vi "NTV_AutoStringArray.vi"(7 "Read(f) Write(t)":bool, 11 "Array":string[](array[string])) -> (3 "Array 2":string[](array[string]))   [LabVIEW 2020]
uses:
  <vilib>/Rock Robotics/Network Tables/NT Read String Array.vi
  <vilib>/Rock Robotics/Network Tables/NT Write String Array.vi
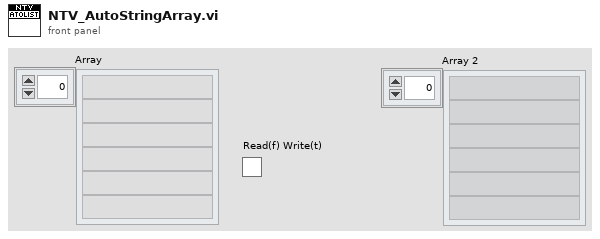
[diagram p1: front panel]
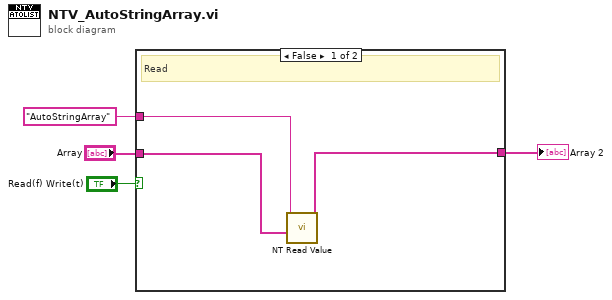
[diagram p0: block diagram]
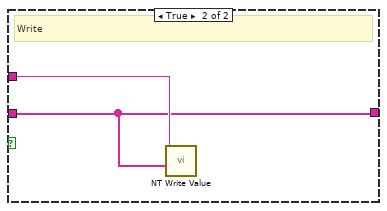
[diagram p2: hidden frame]
diagram:
  n1 = case shown="False" "Read(f) Write(t)" {
    tunnel: "Array" -> [w6 w8]
    tunnel: "AutoStringArray" ("Name") -> [w7 w9]
    tunnel: [w5 w8] -> w1
    frame False {
      # "Read"
      n2 = call-poly <vilib>:"NT Read Value.vi"("default value"=w6, "name"=w7) -> ("value"=w5:string[])  [unwired: 7 in, 2 out]
    }
    frame True {
      # "Write"
      n3 = call-poly <vilib>:"NT Write Value.vi"("value"=w8, "name"=w9) -> ()  [unwired: 9 in, 1 out]
    }
  }
  "Array 2" <- w1
